vi "SPI_Send.vi"() -> ()   [LabVIEW 2018]
uses:
  <userlib>/SPI Digital Waveform/SDW.lvlib
  <userlib>/SPI Digital Waveform/_Polymorphics/Init-Preallocate-fmt1.vi
  <userlib>/SPI Digital Waveform/_Polymorphics/Init-Preallocate-fmt0.vi
  <userlib>/SPI Digital Waveform/_Polymorphics/Swap-U16-fmt1.vi
  <userlib>/SPI Digital Waveform/_Polymorphics/Close-fmt1.vi
  <userlib>/SPI Digital Waveform/_Polymorphics/Send-U16-fmt0.vi
  <userlib>/SPI Digital Waveform/_Polymorphics/Close-fmt0.vi
  <userlib>/SPI Digital Waveform/_Typedefs/Timing-ns.ctl
  <userlib>/SPI Digital Waveform/_Typedefs/Bus config.ctl
panel:
  in  "CPHA":bool
  out "Compare bit locations":u64[](array[numeric])=[20, 70, 120, 170, 220, 270, 320, 370, 420, 470, 520, 570, 620, 670, 720, 770]
  out "SPI Waveform":digitalwaveform(graph)={"t0"=timestamp(0 s since 1904-01-01), "dt"=0.0, "Y"={"transitions"=[], "data"=[]}, "error"={"status"=FALSE, "code"=37421928, "source"=""}}
  in  "Sample quantum":i32=2 min=1
  in  "Slave address":u8
  in  "Expected MISO data":u16=52428 format="%.0x"
  in  "MOSI data":u16=43690 format="%.0x"
  out "Coerced SPI timing":T1={"MOSI Setup"=99.99999999999999, "SCLK Freq"=2000000.0, "SCLK Hold"=199.99999999999997, "CS Lead"=99.99999999999999, "CS Trail"=99.99999999999999, "CS Idle"=199.99999999999997} {"CS Idle" format="%#_6p"; "CS Trail" format="%#_6p"; "SCLK Hold" format="%#_6p"; "SCLK Freq" format="%#_6p"}
  in  "Samples to allocate":i32=100000 format="%.0p"
  in  "Bus configuration":T2={"CPOL"=FALSE, "CS active state"=FALSE, "# of slaves"=1}
  in  "Sample rate":dbl=100000000.0 format="%#_6p"
  in  "SPI timing (ns)":T1={"MOSI Setup"=100.0, "SCLK Freq"=2000000.0, "SCLK Hold"=200.0, "CS Lead"=100.0, "CS Trail"=100.0, "CS Idle"=200.0} {"CS Idle" format="%#_6p"; "CS Trail" format="%#_6p"; "SCLK Hold" format="%#_6p"; "SCLK Freq" format="%#_6p"}
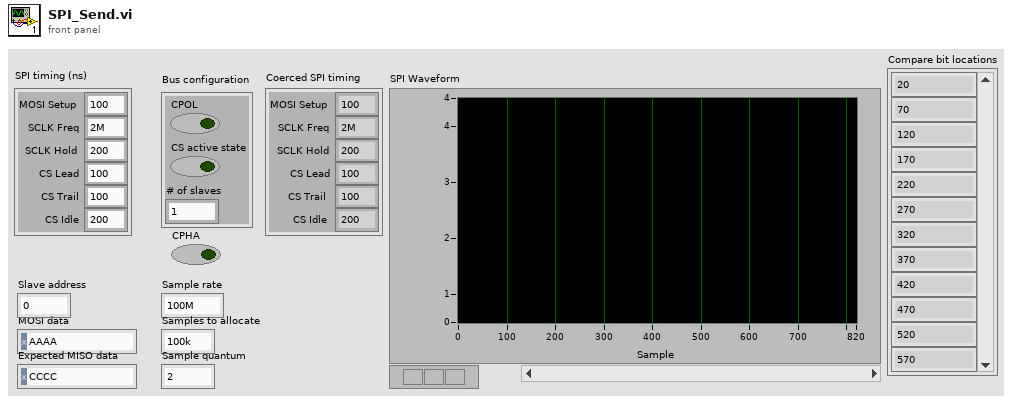
[diagram p1: front panel]
types:
  T1 = typedef "SDW.lvlib/Timing-ns.ctl" = cluster{"MOSI Setup":dbl, "SCLK Freq":dbl, "SCLK Hold":dbl, "CS Lead":dbl, "CS Trail":dbl, "CS Idle":dbl}
  T2 = typedef "SDW.lvlib/Bus config.ctl" = cluster{"CPOL":bool, "CS active state":bool, "# of slaves":u8}
  T3 = typedef "SDW.lvlib/Waveform info-fmt0.ctl" = cluster{"Data":u8[][], "Last sample":u8[], "Preallocated":bool, "Sample offset":u64, "Compare offset":u64, "Compare locations":u64[], "SPI timing (ticks)":T4, "CPOL":bool, "CS active":bool}
  T4 = typedef "SDW.lvlib/Timing-ticks-fmt0.ctl" = cluster{"Idle":i32, "CSa-SU":i32, "SU-SCLKa":i32, "SCLKa-SCLKd":i32, "SCLKd-SU":i32, "SCLKd-CSd":i32}
  T5 = typedef "SDW.lvlib/Waveform info-fmt1.ctl" = cluster{"Data":u8[][], "Last sample":u8[], "Preallocated":bool, "Sample offset":u64, "Compare offset":u64, "Compare locations":u64[], "SPI timing (ticks)":T6, "CPOL":bool, "CS active":bool, "<fmt1 dummy>":bool}
  T6 = typedef "SDW.lvlib/Timing-ticks-fmt1.ctl" = cluster{"Idle":i32, "CSa-SCLKa":i32, "SCLKa-SU":i32, "SU-SCLKd":i32, "SCLKd-SCLKa":i32, "SCLKd-CSd":i32}
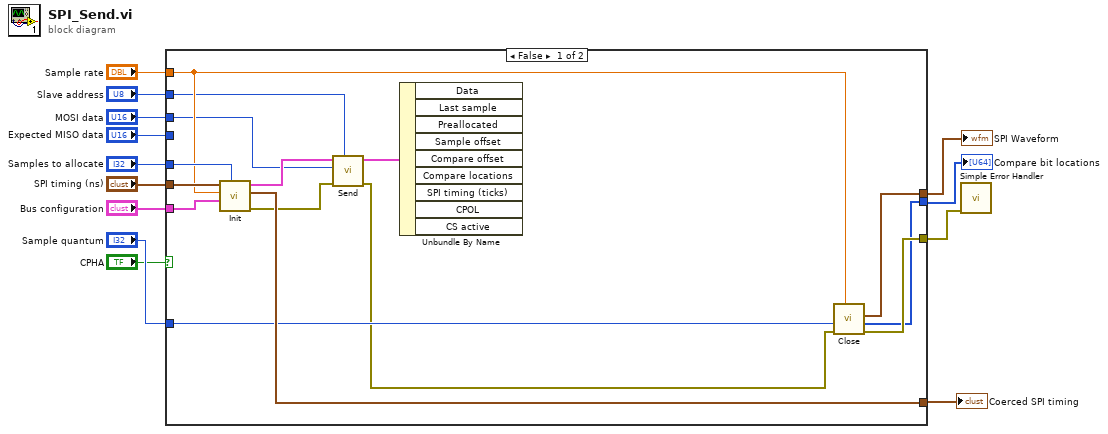
[diagram p0: block diagram]
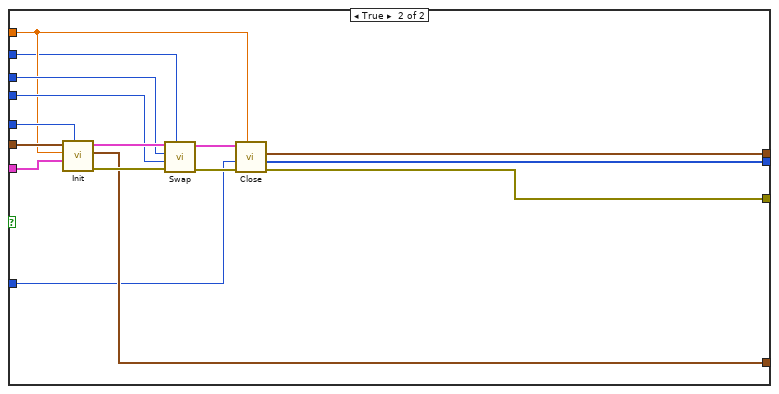
[diagram p2: hidden frame]
diagram:
  n1 = case shown="False" "CPHA" {
    tunnel: "Bus configuration" -> [w28 w40]
    tunnel: "SPI timing (ns)" -> [w27 w39]
    tunnel: "Samples to allocate" -> [w26 w38]
    tunnel: [w25 w37] -> w10
    tunnel: "MOSI data" -> [w17 w36]
    tunnel: "Expected MISO data" -> [_ w35]
    tunnel: "Slave address" -> [w19 w29]
    tunnel: "Sample rate" -> [w24 w34]
    tunnel: "Sample quantum" -> [w23 w33]
    tunnel: [w22 w32] -> w4
    tunnel: [w21 w31] -> w3
    tunnel: [w20 w30] -> w2
    frame False {
      n2 = call-poly <userlib>:"Init.vi"("Samples to allocate"=w26, "Bus configuration"=w28, "Sample rate"=w24, "SPI timing (ns)"=w27) -> ("error out"=w16:errorcluster, "Coerced SPI timing"=w25:T1, "SPI waveform info"=w18:T3)  [unwired: 1 in, 4 out]
      n3 = call-poly <userlib>:"Send.vi"("Slave address"=w19, "error in (no error)"=w16, "MOSI data"=w17, "SPI waveform info"=w18) -> ("error out"=w15:errorcluster, "SPI waveform info out"=w14:T3)  [unwired: 6 in]
      n4 = Unbundle By Name(w14) -> ()  [unwired: 9 out]
      n5 = call-poly <userlib>:"Close.vi"("Sample rate"=w24, "error in (no error)"=w15, "Sample quantum (min 1)"=w23) -> ("error out"=w21:errorcluster, "Compare bit locations"=w20:u64[], "Dig waveform out"=w22:digitalwaveform)  [unwired: 1 in, 5 out]
    }
    frame True {
      n6 = call-poly <userlib>:"Init.vi"("Samples to allocate"=w38, "Bus configuration"=w40, "Sample rate"=w34, "SPI timing (ns)"=w39) -> ("error out"=w42:errorcluster, "Coerced SPI timing"=w37:T1, "SPI waveform info"=w44:T5)  [unwired: 1 in, 4 out]
      n7 = call-poly <userlib>:"Swap.vi"("Slave address"=w29, "error in (no error)"=w42, "Expected MISO data"=w35, "MOSI data"=w36, "SPI waveform info"=w44) -> ("error out"=w41:errorcluster, "SPI waveform info out"=w43:T5)  [unwired: 1 in, 4 out]
      n8 = call-poly <userlib>:"Close.vi"("Sample rate"=w34, "error in (no error)"=w41, "Sample quantum (min 1)"=w33, "SPI waveform info"=w43) -> ("error out"=w31:errorcluster, "Compare bit locations"=w30:u64[], "Dig waveform out"=w32:digitalwaveform)  [unwired: 5 out]
    }
  }
  "Coerced SPI timing" <- w10
  "SPI Waveform" <- w4
  "Compare bit locations" <- w2
  n9 = call <vilib>:"Simple Error Handler.vi"("error in (no error)"=w3) -> ()  [unwired: 1 in, 8 out]
